vi "LV SCISDK Init Lib.vi"() -> (3 "function return":u64)   [LabVIEW 2021, in "SciSDK_Labview.lvlib"]
doc: "You need this VI to allocate memory for a SciSDK library instance"
uses:
  SciSDK_Labview.lvlib
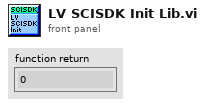
[diagram p1: front panel]
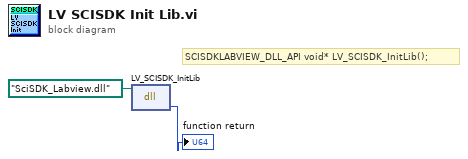
[diagram p0: block diagram]
diagram:
  # "SCISDKLABVIEW_DLL_API void* LV_SCISDK_InitLib();"
  n1 = dll-call lib="C:/git/scisdk/bin/x64/Release/SciSDK_Labview.dll" fn="LV_SCISDK_InitLib"(path in=path "SciSDK_Labview.dll") -> ("return type"=→"function return":u64)  [unwired: 2 in, 2 out]
